vi "Set Light HSB By Name.vi"(7 "Name":string, 8 "Error In":errorcluster, 10 "HSB":T1={"Hue"=0, "Saturation"=255, "Brightness"=255}, 11 "Hue Config":T2) -> (0 "Error Out":errorcluster, 3 "Hue Config":T2)   [LabVIEW 2013, in "LMH-Hue.lvlib"]
uses:
  LMH-Hue.lvlib
  Type Defs/Hue Ref.ctl
  <vilib>/httpClient/ClientHandle.ctl
  Type Defs/Light.ctl
  Type Defs/HSB.ctl
  <vilib>/httpClient/LabVIEWHTTPClient.lvlib
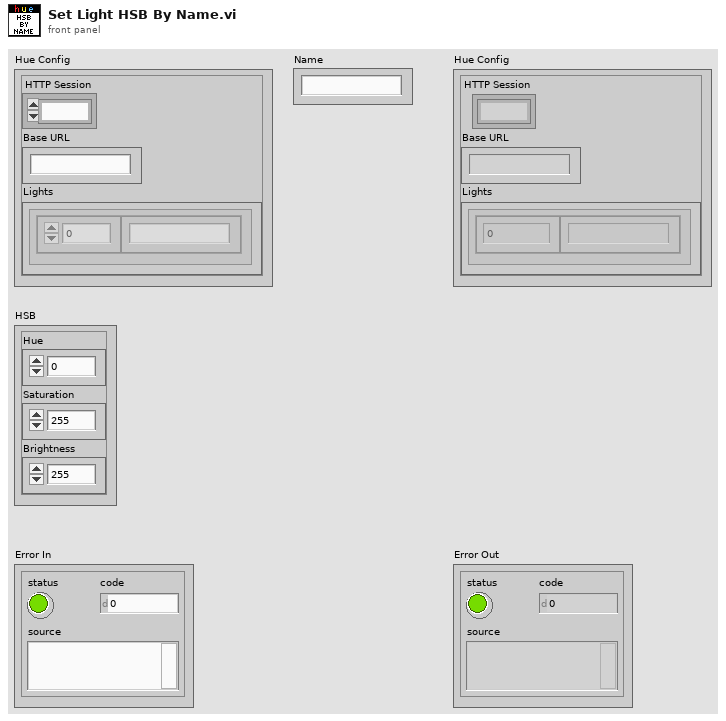
[diagram p1: front panel]
types:
  T1 = typedef "LMH-Hue.lvlib/HSB.ctl" = cluster{"Hue":u16, "Saturation":u8, "Brightness":u8}
  T2 = typedef "LMH-Hue.lvlib/Hue Ref.ctl" = cluster{"HTTP Session":T3, "Base URL":string, "Lights":T4[]}
  T3 = typedef "LabVIEWHTTPClient.lvlib/ClientHandle.ctl" = refnum<k1>
  T4 = typedef "LMH-Hue.lvlib/Light.ctl" = cluster{"ID":i32, "Name":string}
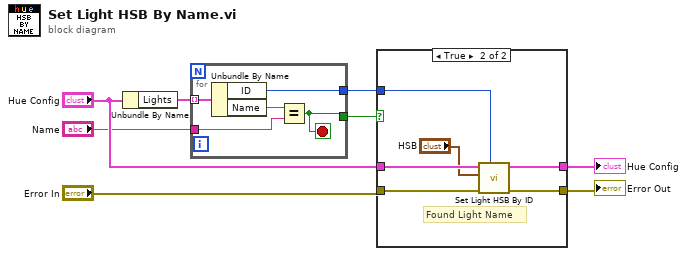
[diagram p0: block diagram]
diagram:
  n1 = Unbundle By Name("Hue Config") -> ("Lights"=w5:T4[])
  n2 = for {
    tunnel: w5 -> [w13] mode=indexing
    tunnel: [w11] -> w1
    tunnel: "Name" -> [w10]
    tunnel: [w9] -> w3
    stop <- w9 stop-if-true
    n3 = Unbundle By Name(w13) -> ("ID"=w11:i32, "Name"=w12:string)
    n4 = Equal?(x=w12, y=w10) -> (x = y?=w9:bool)
  }
  n5 = case shown="True" w3 {
    tunnel: "Error In" -> [w15 w21]
    tunnel: [w14 w20] -> w7
    tunnel: "Hue Config" -> [w14 w19]
    tunnel: [w15 w18] -> w2
    tunnel: w1 -> [_ w17]
    frame False {
      # "No Light By That Name\nThrow Error"
    }
    frame True {
      # "Found Light Name"
      n6 = call "Set Light HSB By ID.vi"("ID"=w17, "Error In"=w21, "HSB"="HSB", "Hue Config"=w19) -> ("Error Out"=w18:errorcluster, "Hue Config"=w20:T2)  [unwired: 6 in]
    }
  }
  "Error Out" <- w2
  "Hue Config" <- w7
